vi "Execute Query.vi"(8 "error in (no error)":errorcluster, 10 "SQL query":string, 11 "SQLite Database in":refnum<class "SQLite Database.lvclass">) -> (0 "error out":errorcluster, 3 "SQLite Database out":refnum<class "SQLite Database.lvclass">)   [LabVIEW 2023, in "HardwareAbstractionLayer_LVOOP.lvlib" / "SQLite Database.lvclass"]
uses:
  SQLite Database.lvclass
  Database.lvclass
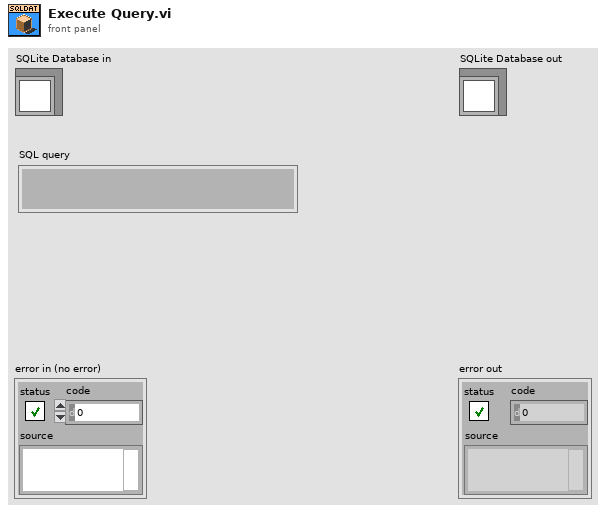
[diagram p1: front panel]
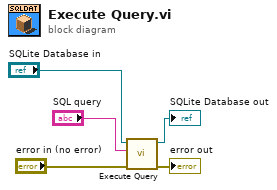
[diagram p0: block diagram]
diagram:
  n1 = call-parent "Execute Query.vi"("error in (no error)"="error in (no error)", "SQL query"="SQL query", "Database in"="SQLite Database in") -> ("error out"=→"error out":errorcluster, "Database out"=→"SQLite Database out":refnum<class "SQLite Database.lvclass">)  [unwired: 7 in]
